vi "Print.vi"(8 "error in":errorcluster, 10 "Anything In":variant, 11 "Printer in":refnum<class "Printer.lvclass">) -> (0 "error out":errorcluster, 2 "Printed String":string, 3 "Printer out":refnum<class "Printer.lvclass">)   [LabVIEW 2020, in "Approval Tests.lvlib" / "Printer.lvclass"]
uses:
  Printer.lvclass
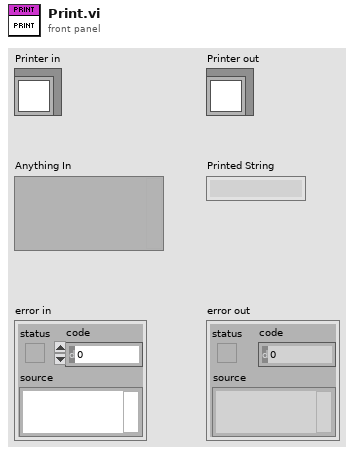
[diagram p1: front panel]
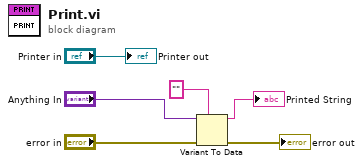
[diagram p0: block diagram]
diagram:
  n1 = Variant To Data(error in="error in", type="", Variant="Anything In") -> (data=→"Printed String":string, error out=→"error out":errorcluster)
  "Printer out" <- "Printer in"
